vi "Get Factory Pattern.vi"() -> (3 "Classes":string[](array[string]))   [LabVIEW 2020, in "FGen.lvlib"]
uses:
  FGen.lvlib
  Generador/Generador.lvclass
  GeneradorAmplificado/GeneradorAmplificado.lvclass
  C:/Users/HP/Documents/7mo/Instrumentacion/Examen_2doParcial/IV2Parcial-develop/Libraries/FGen/Generador/Generador.lvclass
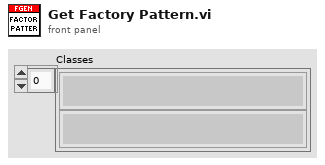
[diagram p1: front panel]
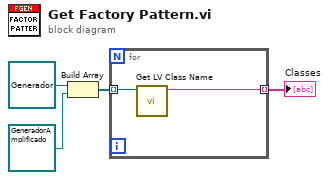
[diagram p0: block diagram]
diagram:
  n1 = Build Array(refnum<class "Generador.lvclass"> refnum ("FGen.lvlib:Generator"), refnum<class "GeneradorAmplificado.lvclass"> refnum ("FGen.lvlib:GeneradorAmplificado.lvclass")) -> (w4:refnum<class "Generador.lvclass">[])
  n2 = for {
    tunnel: w4 -> [w6] mode=indexing
    tunnel: [w5] -> w3 mode=indexing
    n3 = call <vilib>:"Get LV Class Name.vi"("object"=w6) -> ("class name"=w5:string)  [unwired: 9 in, 1 out]
  }
  "Classes" <- w3
